vi "App - analyze RUS V6.vi"() -> ()   [LabVIEW 2015] (continued)
"phase"=3.0483689500573607, "Q"=31924.655099131884, "Norm  Ampl"=0.0072958662795648815, "z (inf)"=-0.1566571183741111-0.36129377749056607i, "4corners"={"z (-pi/2)"=-0.47329377749056606+0.020657118374111084i, "z(inf)"=-0.1566571183741111-0.36129377749056607i, "z (pi/2)"=0.22529377749056606-0.044657118374111106i, "z center"=-0.124-0.01200000000000001i, "z(0)"=-0.09134288162588891+0.33729377749056605i, "radius"=0.35081708962667396}}, "timestamp(min)"=939.1499999985099, "timestamp"=timestamp(3493784170 s since 1904-01-01), "Magn Field(T)"=0.0}, {"temperature"=73.253, "lorentzian"={"Amplitude"=0.00019495658027975842, "omega(0)"=663.9104025268014, "Gamma"=0.023023745131469733, "phase"=3.131685954619118, "Q"=28835.89957827249, "Norm  Ampl"=0.011117450646524998, "z (inf)"=0.007216441342229177-0.49484521216169003i, "4corners"={"z (-pi/2)"=-0.47084521216169-0.007216441342229177i, "z(inf)"=0.007216441342229177-0.49484521216169003i, "z (pi/2)"=0.49484521216169003-0.016783558657770845i, "z center"=0.01200000000000001-0.01200000000000001i, "z(0)"=0.016783558657770845+0.47084521216169i, "radius"=0.48286890699329543}}, "timestamp(min)"=940.4833333343267, "timestamp"=timestamp(3493784250 s since 1904-01-01), "Magn Field(T)"=0.0}, {"temperature"=73.185, "lorentzian"={"Amplitude"=0.00017519026701110808, "omega(0)"=663.8919973297286, "Gamma"=0.020890470676565787, "phase"=3.0576685573030025, "Q"=31779.657223063903, "Norm  Ampl"=0.0069963159787889955, "z (inf)"=-0.16807358892896002-0.33772594277637363i, "4corners"={"z (-pi/2)"=-0.47372594277637364+0.02407358892896001i, "z(inf)"=-0.16807358892896002-0.33772594277637363i, "z (pi/2)"=0.19372594277637362-0.03207358892896002i, "z center"=-0.14-0.0040000000000000036i, "z(0)"=-0.11192641107104+0.3297259427763736i, "radius"=0.3349046599815112}}, "timestamp(min)"=941.8000000044703, "timestamp"=timestamp(3493784329 s since 1904-01-01), "Magn Field(T)"=0.0}, {"temperature"=73.117, "lorentzian"={"Amplitude"=0.00017435824596551483, "omega(0)"=663.8725802754554, "Gamma"=0.02068445495091924, "phase"=3.0424021763685554, "Q"=32095.24166098233, "Norm  Ampl"=0.00621721189787517, "z (inf)"=-0.2017652258022671-0.3030966975685784i, "4corners"={"z (-pi/2)"=-0.47109669756857836+0.02576522580226712i, "z(inf)"=-0.2017652258022671-0.3030966975685784i, "z (pi/2)"=0.1270966975685784-0.033765225802267124i, "z center"=-0.172-0.0040000000000000036i, "z(0)"=-0.14223477419773287+0.29509669756857837i, "radius"=0.30057412257792515}}, "timestamp(min)"=943.1166666671634, "timestamp"=timestamp(3493784408 s since 1904-01-01), "Magn Field(T)"=0.0}, {"temperature"=73.048, "lorentzian"={"Amplitude"=0.00017676330015604157, "omega(0)"=663.8531342977661, "Gamma"=0.02121284701140279, "phase"=3.0670891125022886, "Q"=31294.86268113457, "Norm  Ampl"=0.007605974320098498, "z (inf)"=-0.15068891735183343-0.361560422826347i, "4corners"={"z (-pi/2)"=-0.481560422826347+0.02268891735183344i, "z(inf)"=-0.15068891735183343-0.361560422826347i, "z (pi/2)"=0.23356042282634698-0.030688917351833447i, "z center"=-0.124-0.0040000000000000036i, "z(0)"=-0.09731108264816656+0.353560422826347i, "radius"=0.3585550923933016}}, "timestamp(min)"=944.4500000029802, "timestamp"=timestamp(3493784488 s since 1904-01-01), "Magn Field(T)"=0.0}, {"temperature"=72.978, "lorentzian"={"Amplitude"=0.00018345336821167508, "omega(0)"=663.834753319743, "Gamma"=0.022043405813372347, "phase"=3.126951039938785, "Q"=30114.890545499835, "Norm  Ampl"=0.01041417114121995, "z (inf)"=-0.018917026509175042-0.48438865766564027i, "4corners"={"z (-pi/2)"=-0.48438865766564027-0.00508297349082498i, "z(inf)"=-0.018917026509175042-0.48438865766564027i, "z (pi/2)"=0.46038865766564024-0.018917026509175042i, "z center"=-0.01200000000000001-0.01200000000000001i, "z(0)"=-0.00508297349082498+0.46038865766564024i, "radius"=0.47243929678517865}}, "timestamp(min)"=945.7666666656733, "timestamp"=timestamp(3493784567 s since 1904-01-01), "Magn Field(T)"=0.0}, {"temperature"=72.911, "lorentzian"={"Amplitude"=0.0001551220169346823, "omega(0)"=663.8174664217973, "Gamma"=0.018764064565812026, "phase"=3.0713605879648487, "Q"=35377.06151530023, "Norm  Ampl"=0.008325788969481407, "z (inf)"=-0.06713700481821767-0.4546153898054041i, "4corners"={"z (-pi/2)"=-0.4786153898054041+0.01913700481821769i, "z(inf)"=-0.06713700481821767-0.4546153898054041i, "z (pi/2)"=0.4066153898054041-0.04313700481821771i, "z center"=-0.035999999999999976-0.01200000000000001i, "z(0)"=-0.004862995181782275+0.4306153898054041i, "radius"=0.44370924755028435}}, "timestamp(min)"=947.1000000014901, "timestamp"=timestamp(3493784647 s since 1904-01-01), "Magn Field(T)"=0.0}, {"temperature"=72.846, "lorentzian"={"Amplitude"=0.0001555991138381181, "omega(0)"=663.7976768196731, "Gamma"=0.018698213519798536, "phase"=3.053995868272443, "Q"=35500.59347203482, "Norm  Ampl"=0.007017682837638503, "z (inf)"=-0.1408341852026201-0.3778740073328248i, "4corners"={"z (-pi/2)"=-0.48187400733282476+0.028834185202620086i, "z(inf)"=-0.1408341852026201-0.3778740073328248i, "z (pi/2)"=0.2658740073328248-0.03683418520262009i, "z center"=-0.10799999999999998-0.0040000000000000036i, "z(0)"=-0.0751658147973799+0.3698740073328248i, "radius"=0.37531301213390544}}, "timestamp(min)"=948.4166666641831, "timestamp"=timestamp(3493784726 s since 1904-01-01), "Magn Field(T)"=0.0}, {"temperature"=72.777, "lorentzian"={"Amplitude"=0.00015084357573425, "omega(0)"=663.7786903386511, "Gamma"=0.017971078540124134, "phase"=3.0293798474399702, "Q"=36935.94064800443, "Norm  Ampl"=0.005825438199226138, "z (inf)"=-0.19229819911547524-0.3261175918457008i, "4corners"={"z (-pi/2)"=-0.47811759184570085+0.032298199115475205i, "z(inf)"=-0.19229819911547524-0.3261175918457008i, "z (pi/2)"=0.1661175918457008-0.04029819911547521i, "z center"=-0.15600000000000003-0.0040000000000000036i, "z(0)"=-0.11970180088452481+0.3181175918457008i, "radius"=0.32415629291361936}}, "timestamp(min)"=949.7333333343267, "timestamp"=timestamp(3493784805 s since 1904-01-01), "Magn Field(T)"=0.0}, {"temperature"=72.707, "lorentzian"={"Amplitude"=0.00014939699892849853, "omega(0)"=663.7592398477731, "Gamma"=0.017930072072597437, "phase"=3.031276824620436, "Q"=37019.329156082844, "Norm  Ampl"=0.006595607315274654, "z (inf)"=-0.15649760753219724-0.3696156584222518i, "4corners"={"z (-pi/2)"=-0.4816156584222518+0.036497607532197246i, "z(inf)"=-0.15649760753219724-0.3696156584222518i, "z (pi/2)"=0.2496156584222518-0.04449760753219725i, "z center"=-0.11599999999999999-0.0040000000000000036i, "z(0)"=-0.07550239246780274+0.3616156584222518i, "radius"=0.36785169008632895}}, "timestamp(min)"=951.0666666701436, "timestamp"=timestamp(3493784885 s since 1904-01-01), "Magn Field(T)"=0.0}, {"temperature"=72.643, "lorentzian"={"Amplitude"=0.00017077398769670094, "omega(0)"=663.738826060015, "Gamma"=0.020607074561124927, "phase"=3.0746062633397298, "Q"=32209.269884050045, "Norm  Ampl"=0.0086712605421239, "z (inf)"=-0.08816615902804703-0.43184674010553753i, "4corners"={"z (-pi/2)"=-0.4798467401055375+0.01616615902804702i, "z(inf)"=-0.08816615902804703-0.43184674010553753i, "z (pi/2)"=0.3598467401055375-0.040166159028047044i, "z center"=-0.06-0.01200000000000001i, "z(0)"=-0.031833840971952965+0.4078467401055375i, "radius"=0.4207904676815291}}, "timestamp(min)"=952.3833333328366, "timestamp"=timestamp(3493784964 s since 1904-01-01), "Magn Field(T)"=0.0}, {"temperature"=72.574, "lorentzian"={"Amplitude"=0.00015213404269060979, "omega(0)"=663.7213392465111, "Gamma"=0.01837305169166479, "phase"=3.035741424854037, "Q"=36124.719528635425, "Norm  Ampl"=0.006585091339083578, "z (inf)"=-0.16186736619318068-0.3604042931463336i, "4corners"={"z (-pi/2)"=-0.4804042931463336+0.033867366193180676i, "z(inf)"=-0.16186736619318068-0.3604042931463336i, "z (pi/2)"=0.2324042931463336-0.04186736619318068i, "z center"=-0.124-0.0040000000000000036i, "z(0)"=-0.08613263380681932+0.3524042931463336i, "radius"=0.3584103201577016}}, "timestamp(min)"=953.7000000029802, "timestamp"=timestamp(3493785043 s since 1904-01-01), "Magn Field(T)"=0.0}, {"temperature"=72.507, "lorentzian"={"Amplitude"=0.0001470715960104401, "omega(0)"=663.7025470782887, "Gamma"=0.01782665731894476, "phase"=3.04998161802813, "Q"=37230.90286662762, "Norm  Ampl"=0.006247681308114839, "z (inf)"=-0.16406188847504188-0.35299883018424616i, "4corners"={"z (-pi/2)"=-0.48099883018424616+0.028061888475041874i, "z(inf)"=-0.16406188847504188-0.35299883018424616i, "z (pi/2)"=0.21699883018424615-0.03606188847504188i, "z center"=-0.132-0.0040000000000000036i, "z(0)"=-0.09993811152495813+0.34499883018424615i, "radius"=0.35046846956974365}}, "timestamp(min)"=955.0333333313465, "timestamp"=timestamp(3493785123 s since 1904-01-01), "Magn Field(T)"=0.0}, {"temperature"=72.439, "lorentzian"={"Amplitude"=0.0001556972144457539, "omega(0)"=663.6810373710007, "Gamma"=0.0190413758844246, "phase"=3.0950823081436862, "Q"=34854.67864293758, "Norm  Ampl"=0.006603870241185977, "z (inf)"=-0.15612475706680048-0.35044181083865616i, "4corners"={"z (-pi/2)"=-0.4864418108386562+0.012124757066800471i, "z(inf)"=-0.15612475706680048-0.35044181083865616i, "z (pi/2)"=0.20644181083865615-0.02012475706680048i, "z center"=-0.14-0.0040000000000000036i, "z(0)"=-0.12387524293319954+0.34244181083865616i, "radius"=0.3468168624614878}}, "timestamp(min)"=956.3500000014901, "timestamp"=timestamp(3493785202 s since 1904-01-01), "Magn Field(T)"=0.0}, {"temperature"=72.371, "lorentzian"={"Amplitude"=0.0001507592891099395, "omega(0)"=663.6638983583827, "Gamma"=0.01869568647863634, "phase"=3.0980461327038666, "Q"=35498.23640425052, "Norm  Ampl"=0.006397856598824616, "z (inf)"=-0.14689735890560787-0.35388589109003726i, "4corners"={"z (-pi/2)"=-0.47388589109003726+0.002897358905607862i, "z(inf)"=-0.14689735890560787-0.35388589109003726i, "z (pi/2)"=0.20988589109003725-0.026897358905607884i, "z center"=-0.132-0.01200000000000001i, "z(0)"=-0.11710264109439214+0.32988589109003724i, "radius"=0.3422103064327422}}, "timestamp(min)"=957.683333337307, "timestamp"=timestamp(3493785282 s since 1904-01-01), "Magn Field(T)"=0.0}, {"temperature"=72.308, "lorentzian"={"Amplitude"=0.00016230426236795705, "omega(0)"=663.6439303978735, "Gamma"=0.01982415794364744, "phase"=3.131202541165063, "Q"=33476.5255747236, "Norm  Ampl"=0.008567093112471861, "z (inf)"=-0.05649004993272625-0.4441308735094935i, "4corners"={"z (-pi/2)"=-0.48413087350949346-0.00750995006727375i, "z(inf)"=-0.05649004993272625-0.4441308735094935i, "z (pi/2)"=0.3801308735094935-0.01649004993272627i, "z center"=-0.05199999999999999-0.01200000000000001i, "z(0)"=-0.04750995006727373+0.42013087350949346i, "radius"=0.4321541997811386}}, "timestamp(min)"=959.0, "timestamp"=timestamp(3493785361 s since 1904-01-01), "Magn Field(T)"=0.0}, {"temperature"=72.238, "lorentzian"={"Amplitude"=0.0001587208237648037, "omega(0)"=663.6241437684071, "Gamma"=0.018918376740188685, "phase"=3.0783676700778537, "Q"=35078.281444657834, "Norm  Ampl"=0.006359561424550766, "z (inf)"=-0.16123941943617293-0.34748622561900455i, "4corners"={"z (-pi/2)"=-0.47548622561900455+0.009239419436172912i, "z(inf)"=-0.16123941943617293-0.34748622561900455i, "z (pi/2)"=0.19548622561900453-0.03323941943617294i, "z center"=-0.14-0.01200000000000001i, "z(0)"=-0.11876058056382709+0.32348622561900453i, "radius"=0.33615788034504157}}, "timestamp(min)"=960.3166666701436, "timestamp"=timestamp(3493785440 s since 1904-01-01), "Magn Field(T)"=0.0}, {"temperature"=72.173, "lorentzian"={"Amplitude"=0.00014945097138632582, "omega(0)"=663.6053258833265, "Gamma"=0.017943141405183435, "phase"=3.0710983273781256, "Q"=36983.78733679396, "Norm  Ampl"=0.006165904771094313, "z (inf)"=-0.1562043116839784-0.35478225857476353i, "4corners"={"z (-pi/2)"=-0.4747822585747635+0.012204311683978373i, "z(inf)"=-0.1562043116839784-0.35478225857476353i, "z (pi/2)"=0.21078225857476351-0.03620431168397839i, "z center"=-0.132-0.01200000000000001i, "z(0)"=-0.10779568831602163+0.3307822585747635i, "radius"=0.3436357453724964}}, "timestamp(min)"=961.6499999985099, "timestamp"=timestamp(3493785520 s since 1904-01-01), "Magn Field(T)"=0.0}, {"temperature"=72.106, "lorentzian"={"Amplitude"=0.00014166531123358068, "omega(0)"=663.5880613487568, "Gamma"=0.017621215492130873, "phase"=3.063673431163844, "Q"=37658.47263176006, "Norm  Ampl"=0.007707115263841109, "z (inf)"=-0.07804560451196209-0.45604997580422607i, "4corners"={"z (-pi/2)"=-0.48004997580422604+0.014045604511962087i, "z(inf)"=-0.07804560451196209-0.45604997580422607i, "z (pi/2)"=0.39204997580422607-0.05404560451196212i, "z center"=-0.043999999999999984-0.020000000000000018i, "z(0)"=-0.009954395488037879+0.41604997580422604i, "radius"=0.43737705082165784}}, "timestamp(min)"=962.9666666686535, "timestamp"=timestamp(3493785599 s since 1904-01-01), "Magn Field(T)"=0.0}, {"temperature"=72.039, "lorentzian"={"Amplitude"=0.00010361030809420268, "omega(0)"=663.5698546355719, "Gamma"=0.016439285091381955, "phase"=3.1094946906609193, "Q"=40364.885148408204, "Norm  Ampl"=0.005333823694357822, "z (inf)"=-0.1584125865349883-0.38428881406653514i, "4corners"={"z (-pi/2)"=-0.47228881406653517-0.04958741346501172i, "z(inf)"=-0.1584125865349883-0.38428881406653514i, "z (pi/2)"=0.17628881406653513-0.07041258653498828i, "z center"=-0.14800000000000002-0.06i, "z(0)"=-0.13758741346501174+0.26428881406653515i, "radius"=0.32445593982392806}}, "timestamp(min)"=964.2833333313465, "timestamp"=timestamp(3493785678 s since 1904-01-01), "Magn Field(T)"=0.0}, {"temperature"=71.974, "lorentzian"={"Amplitude"=0.0001353918285003591, "omega(0)"=663.5515429002106, "Gamma"=0.016337688977960896, "phase"=3.1152659157247515, "Q"=40614.773839514506, "Norm  Ampl"=0.0059967070933330206, "z (inf)"=-0.11766204581152509-0.37892025850284383i, "4corners"={"z (-pi/2)"=-0.4749202585028438-0.0023379541884749073i, "z(inf)"=-0.11766204581152509-0.37892025850284383i, "z (pi/2)"=0.25892025850284384-0.021662045811525116i, "z center"=-0.10799999999999998-0.01200000000000001i, "z(0)"=-0.09833795418847488+0.3549202585028438i, "radius"=0.36704745092298047}}, "timestamp(min)"=965.6166666671634, "timestamp"=timestamp(3493785758 s since 1904-01-01), "Magn Field(T)"=0.0}, {"temperature"=71.908, "lorentzian"={"Amplitude"=0.00020447876795810522, "omega(0)"=663.5338391109882, "Gamma"=0.024406535860778355, "phase"=3.462541685023603, "Q"=27186.727477261382, "Norm  Ampl"=0.009353380375411984, "z (inf)"=0.028897345607210093-0.415663392708284i, "4corners"={"z (-pi/2)"=-0.45566339270828404-0.1728973456072101i, "z(inf)"=0.028897345607210093-0.415663392708284i, "z (pi/2)"=0.271663392708284+0.06889734560721013i, "z center"=-0.09200000000000003-0.05199999999999999i, "z(0)"=-0.21289734560721013+0.311663392708284i, "radius"=0.3832326073952591}}, "timestamp(min)"=966.933333337307, "timestamp"=timestamp(3493785837 s since 1904-01-01), "Magn Field(T)"=0.0}, {"temperature"=71.842, "lorentzian"={"Amplitude"=0.00020284598772034006, "omega(0)"=663.5159545204048, "Gamma"=0.02385301531569419, "phase"=3.438102919866405, "Q"=27816.858612581433, "Norm  Ampl"=0.010641694016462908, "z (inf)"=0.09435410712337688-0.502667705428403i, "4corners"={"z (-pi/2)"=-0.462667705428403-0.20635410712337687i, "z(inf)"=0.09435410712337688-0.502667705428403i, "z (pi/2)"=0.39066770542840307+0.05435410712337685i, "z center"=-0.035999999999999976-0.07600000000000001i, "z(0)"=-0.16635410712337684+0.35066770542840303i, "radius"=0.4461362169780339}}, "timestamp(min)"=968.2666666656733, "timestamp"=timestamp(3493785917 s since 1904-01-01), "Magn Field(T)"=0.0}, {"temperature"=71.776, "lorentzian"={"Amplitude"=0.0001158178599625776, "omega(0)"=663.4970989685446, "Gamma"=0.017705924903385337, "phase"=3.1260543468802098, "Q"=37473.168026465835, "Norm  Ampl"=0.006876638691775869, "z (inf)"=-0.09003453488478114-0.45633376972380324i, "4corners"={"z (-pi/2)"=-0.47233376972380325-0.06196546511521888i, "z(inf)"=-0.09003453488478114-0.45633376972380324i, "z (pi/2)"=0.3043337697238032-0.07403453488478112i, "z center"=-0.08400000000000002-0.068i, "z(0)"=-0.0779654651152189+0.32033376972380323i, "radius"=0.3883806538940572}}, "timestamp(min)"=969.5833333358169, "timestamp"=timestamp(3493785996 s since 1904-01-01), "Magn Field(T)"=0.0}, {"temperature"=71.708, "lorentzian"={"Amplitude"=0.00014344606787871066, "omega(0)"=663.4769127694987, "Gamma"=0.018079577085066488, "phase"=3.0739753162348773, "Q"=36697.59030577781, "Norm  Ampl"=0.007230938052613988, "z (inf)"=-0.1030229929735954-0.4110366596727773i, "4corners"={"z (-pi/2)"=-0.4750366596727773+0.01502299297359539i, "z(inf)"=-0.1030229929735954-0.4110366596727773i, "z (pi/2)"=0.3230366596727773-0.03902299297359541i, "z center"=-0.07600000000000001-0.01200000000000001i, "z(0)"=-0.04897700702640461+0.3870366596727773i, "radius"=0.3999506193420119}}, "timestamp(min)"=970.8999999985099, "timestamp"=timestamp(3493786075 s since 1904-01-01), "Magn Field(T)"=0.0}, {"temperature"=71.643, "lorentzian"={"Amplitude"=1.7606488630633843e-05, "omega(0)"=663.4981912028674, "Gamma"=0.002347216628142593, "phase"=2.6632845873121296, "Q"=282674.4592926256, "Norm  Ampl"=0.0022609898934732864, "z (inf)"=-0.0153691348783212-0.3791618846869318i, "4corners"={"z (-pi/2)"=-0.4271618846869317+0.9193691348783213i, "z(inf)"=-0.0153691348783212-0.3791618846869318i, "z (pi/2)"=1.283161884686932+0.03263086512167873i, "z center"=0.42800000000000005+0.476i, "z(0)"=0.8713691348783212+1.3311618846869318i, "radius"=0.9632642621752642}}, "timestamp(min)"=972.2333333343267, "timestamp"=timestamp(3493786155 s since 1904-01-01), "Magn Field(T)"=0.0}, {"temperature"=71.578, "lorentzian"={"Amplitude"=1.4211102692804694e-05, "omega(0)"=663.499400259395, "Gamma"=0.0015188613859837142, "phase"=3.0098558230419314, "Q"=436839.99500037933, "Norm  Ampl"=0.0014038362866800934, "z (inf)"=0.3705916271616414-0.5202603006819091i, "4corners"={"z (-pi/2)"=-0.4242603006819091+0.5174083728383586i, "z(inf)"=0.3705916271616414-0.5202603006819091i, "z (pi/2)"=1.408260300681909+0.2745916271616414i, "z center"=0.492+0.396i, "z(0)"=0.6134083728383586+1.3122603006819091i, "radius"=0.9242688632648837}}, "timestamp(min)"=973.5500000044703, "timestamp"=timestamp(3493786234 s since 1904-01-01), "Magn Field(T)"=0.0}, {"temperature"=71.514, "lorentzian"={"Amplitude"=0.0010685633366742913, "omega(0)"=663.450380905746, "Gamma"=0.15922878254567352, "phase"=4.5585256955829605, "Q"=4166.648581360851, "Norm  Ampl"=0.08739969324990009, "z (inf)"=0.322409387202908+0.12787822949289898i, "4corners"={"z (-pi/2)"=-0.304121770507101-0.330409387202908i, "z(inf)"=0.322409387202908+0.12787822949289898i, "z (pi/2)"=-0.135878229492899+0.754409387202908i, "z center"=-0.21999999999999997+0.21199999999999997i, "z(0)"=-0.762409387202908+0.296121770507101i, "radius"=0.5488938108587886}}, "timestamp(min)"=974.8833333328366, "timestamp"=timestamp(3493786314 s since 1904-01-01), "Magn Field(T)"=0.0}, {"temperature"=71.446, "lorentzian"={"Amplitude"=0.0029607355721983555, "omega(0)"=663.468044758759, "Gamma"=0.47900225843268496, "phase"=-0.5808048204263985, "Q"=1385.104210008641, "Norm  Ampl"=0.30913694678107567, "z (inf)"=0.10211629149371892+0.7595487666345311i, "4corners"={"z (-pi/2)"=0.2875487666345311-0.13411629149371895i, "z(inf)"=0.10211629149371892+0.7595487666345311i, "z (pi/2)"=-0.7915487666345311+0.5741162914937189i, "z center"=-0.252+0.21999999999999997i, "z(0)"=-0.6061162914937189-0.31954876663453113i, "radius"=0.6453768042609745}}, "timestamp(min)"=976.2000000029802, "timestamp"=timestamp(3493786393 s since 1904-01-01), "Magn Field(T)"=0.0}, {"temperature"=71.383, "lorentzian"={"Amplitude"=0.0010611794064622126, "omega(0)"=663.4473219222272, "Gamma"=0.2080875040394991, "phase"=-1.3216612968573798, "Q"=3188.309288366935, "Norm  Ampl"=0.11037021324273609, "z (inf)"=0.31802725973655793+0.294779205449031i, "4corners"={"z (-pi/2)"=-0.06522079455096902-0.3500272597365579i, "z(inf)"=0.31802725973655793+0.294779205449031i, "z (pi/2)"=-0.326779205449031+0.678027259736558i, "z center"=-0.196+0.16400000000000003i, "z(0)"=-0.710027259736558+0.033220794550969046i, "radius"=0.5304028886894891}}, "timestamp(min)"=977.5166666656733, "timestamp"=timestamp(3493786472 s since 1904-01-01), "Magn Field(T)"=0.0}, {"temperature"=71.316, "lorentzian"={"Amplitude"=0.003475248520660529, "omega(0)"=663.321849078867, "Gamma"=0.42900679763503213, "phase"=-1.1532083704249727, "Q"=1546.1802767124755, "Norm  Ampl"=0.3966685315298843, "z (inf)"=0.3771678036337911+0.7869862344056386i, "4corners"={"z (-pi/2)"=-0.09301376559436136-0.43316780363379104i, "z(inf)"=0.3771678036337911+0.7869862344056386i, "z (pi/2)"=-0.8429862344056386+1.257167803633791i, "z center"=-0.46799999999999997+0.41200000000000003i, "z(0)"=-1.313167803633791+0.037013765594361425i, "radius"=0.924620620737439}}, "timestamp(min)"=978.8500000014901, "timestamp"=timestamp(3493786552 s since 1904-01-01), "Magn Field(T)"=0.0}, {"temperature"=71.25, "lorentzian"={"Amplitude"=0.0, "omega(0)"=0.0, "Gamma"=0.0, "phase"=0.0, "Q"=0.0, "Norm  Ampl"=0.0, "z (inf)"=0.0+0.0i, "4corners"={"z (-pi/2)"=0.0+0.0i, "z(inf)"=0.0+0.0i, "z (pi/2)"=0.0+0.0i, "z center"=0.0+0.0i, "z(0)"=0.0+0.0i, "radius"=0.0}}, "timestamp(min)"=980.1666666641831, "timestamp"=timestamp(3493786631 s since 1904-01-01), "Magn Field(T)"=0.0}, {"temperature"=71.184, "lorentzian"={"Amplitude"=0.003475248520660529, "omega(0)"=663.321849078867, "Gamma"=0.42900679763503213, "phase"=-1.1532083704249727, "Q"=1546.1802767124755, "Norm  Ampl"=0.3966685315298843, "z (inf)"=0.3771678036337911+0.7869862344056386i, "4corners"={"z (-pi/2)"=-0.09301376559436136-0.43316780363379104i, "z(inf)"=0.3771678036337911+0.7869862344056386i, "z (pi/2)"=-0.8429862344056386+1.257167803633791i, "z center"=-0.46799999999999997+0.41200000000000003i, "z(0)"=-1.313167803633791+0.037013765594361425i, "radius"=0.924620620737439}}, "timestamp(min)"=981.4833333343267, "timestamp"=timestamp(3493786710 s since 1904-01-01), "Magn Field(T)"=0.0}, {"temperature"=71.122, "lorentzian"={"Amplitude"=0.0, "omega(0)"=0.0, "Gamma"=0.0, "phase"=0.0, "Q"=0.0, "Norm  Ampl"=0.0, "z (inf)"=0.0+0.0i, "4corners"={"z (-pi/2)"=0.0+0.0i, "z(inf)"=0.0+0.0i, "z (pi/2)"=0.0+0.0i, "z center"=0.0+0.0i, "z(0)"=0.0+0.0i, "radius"=0.0}}, "timestamp(min)"=982.8166666701436, "timestamp"=timestamp(3493786790 s since 1904-01-01), "Magn Field(T)"=0.0}, {"temperature"=71.056, "lorentzian"={"Amplitude"=0.0, "omega(0)"=0.0, "Gamma"=0.0, "phase"=0.0, "Q"=0.0, "Norm  Ampl"=0.0, "z (inf)"=0.0+0.0i, "4corners"={"z (-pi/2)"=0.0+0.0i, "z(inf)"=0.0+0.0i, "z (pi/2)"=0.0+0.0i, "z center"=0.0+0.0i, "z(0)"=0.0+0.0i, "radius"=0.0}}, "timestamp(min)"=984.1333333328366, "timestamp"=timestamp(3493786869 s since 1904-01-01), "Magn Field(T)"=0.0}, {"temperature"=70.993, "lorentzian"={"Amplitude"=0.0, "omega(0)"=0.0, "Gamma"=0.0, "phase"=0.0, "Q"=0.0, "Norm  Ampl"=0.0, "z (inf)"=0.0+0.0i, "4corners"={"z (-pi/2)"=0.0+0.0i, "z(inf)"=0.0+0.0i, "z (pi/2)"=0.0+0.0i, "z center"=0.0+0.0i, "z(0)"=0.0+0.0i, "radius"=0.0}}, "timestamp(min)"=985.4666666686535, "timestamp"=timestamp(3493786949 s since 1904-01-01), "Magn Field(T)"=0.0}, {"temperature"=70.928, "lorentzian"={"Amplitude"=0.0, "omega(0)"=0.0, "Gamma"=0.0, "phase"=0.0, "Q"=0.0, "Norm  Ampl"=0.0, "z (inf)"=0.0+0.0i, "4corners"={"z (-pi/2)"=0.0+0.0i, "z(inf)"=0.0+0.0i, "z (pi/2)"=0.0+0.0i, "z center"=0.0+0.0i, "z(0)"=0.0+0.0i, "radius"=0.0}}, "timestamp(min)"=986.7833333313465, "timestamp"=timestamp(3493787028 s since 1904-01-01), "Magn Field(T)"=0.0}, {"temperature"=70.86, "lorentzian"={"Amplitude"=0.0, "omega(0)"=0.0, "Gamma"=0.0, "phase"=0.0, "Q"=0.0, "Norm  Ampl"=0.0, "z (inf)"=0.0+0.0i, "4corners"={"z (-pi/2)"=0.0+0.0i, "z(inf)"=0.0+0.0i, "z (pi/2)"=0.0+0.0i, "z center"=0.0+0.0i, "z(0)"=0.0+0.0i, "radius"=0.0}}, "timestamp(min)"=988.1000000014901, "timestamp"=timestamp(3493787107 s since 1904-01-01), "Magn Field(T)"=0.0}, {"temperature"=70.8, "lorentzian"={"Amplitude"=0.0, "omega(0)"=0.0, "Gamma"=0.0, "phase"=0.0, "Q"=0.0, "Norm  Ampl"=0.0, "z (inf)"=0.0+0.0i, "4corners"={"z (-pi/2)"=0.0+0.0i, "z(inf)"=0.0+0.0i, "z (pi/2)"=0.0+0.0i, "z center"=0.0+0.0i, "z(0)"=0.0+0.0i, "radius"=0.0}}, "timestamp(min)"=989.433333337307, "timestamp"=timestamp(3493787187 s since 1904-01-01), "Magn Field(T)"=0.0}, {"temperature"=70.734, "lorentzian"={"Amplitude"=0.00014741895752361318, "omega(0)"=663.2012958301423, "Gamma"=0.019526191075777525, "phase"=3.133366552808286, "Q"=33964.703779471434, "Norm  Ampl"=0.006276995745365551, "z (inf)"=-0.15864437734220443-0.3334545706341914i, "4corners"={"z (-pi/2)"=-0.47745457063419144-0.009355622657795592i, "z(inf)"=-0.15864437734220443-0.3334545706341914i, "z (pi/2)"=0.1654545706341914-0.01464437734220443i, "z center"=-0.15600000000000003-0.01200000000000001i, "z(0)"=-0.15335562265779562+0.3094545706341914i, "radius"=0.3214654471527855}}, "timestamp(min)"=990.75, "timestamp"=timestamp(3493787266 s since 1904-01-01), "Magn Field(T)"=0.0}, {"temperature"=70.67, "lorentzian"={"Amplitude"=0.0, "omega(0)"=0.0, "Gamma"=0.0, "phase"=0.0, "Q"=0.0, "Norm  Ampl"=0.0, "z (inf)"=0.0+0.0i, "4corners"={"z (-pi/2)"=0.0+0.0i, "z(inf)"=0.0+0.0i, "z (pi/2)"=0.0+0.0i, "z center"=0.0+0.0i, "z(0)"=0.0+0.0i, "radius"=0.0}}, "timestamp(min)"=992.0833333358169, "timestamp"=timestamp(3493787346 s since 1904-01-01), "Magn Field(T)"=0.0}, {"temperature"=70.607, "lorentzian"={"Amplitude"=0.00015328744837051362, "omega(0)"=663.1800332004171, "Gamma"=0.020013063108302323, "phase"=3.144815040514048, "Q"=33137.35781532114, "Norm  Ampl"=0.006378181417753034, "z (inf)"=-0.1629730241332717-0.322699255004469i, "4corners"={"z (-pi/2)"=-0.482699255004469-0.005026975866728277i, "z(inf)"=-0.1629730241332717-0.322699255004469i, "z (pi/2)"=0.15469925500446902-0.00297302413327173i, "z center"=-0.16399999999999998-0.0040000000000000036i, "z(0)"=-0.16502697586672826+0.314699255004469i, "radius"=0.31870090966270304}}, "timestamp(min)"=993.3999999985099, "timestamp"=timestamp(3493787425 s since 1904-01-01), "Magn Field(T)"=0.0}, {"temperature"=70.54, "lorentzian"={"Amplitude"=0.00016009520963442775, "omega(0)"=663.1586234942882, "Gamma"=0.021315116129614096, "phase"=3.2383816283953406, "Q"=31112.128100157555, "Norm  Ampl"=0.00921059739114969, "z (inf)"=-0.01824123099103222-0.4340932765652777i, "4corners"={"z (-pi/2)"=-0.4900932765652777-0.04575876900896778i, "z(inf)"=-0.01824123099103222-0.4340932765652777i, "z (pi/2)"=0.3700932765652777+0.037758769008967775i, "z center"=-0.06-0.0040000000000000036i, "z(0)"=-0.10175876900896777+0.4260932765652777i, "radius"=0.4321157499279571}}, "timestamp(min)"=994.7166666686535, "timestamp"=timestamp(3493787504 s since 1904-01-01), "Magn Field(T)"=0.0}, {"temperature"=70.48, "lorentzian"={"Amplitude"=0.0, "omega(0)"=0.0, "Gamma"=0.0, "phase"=0.0, "Q"=0.0, "Norm  Ampl"=0.0, "z (inf)"=0.0+0.0i, "4corners"={"z (-pi/2)"=0.0+0.0i, "z(inf)"=0.0+0.0i, "z (pi/2)"=0.0+0.0i, "z center"=0.0+0.0i, "z(0)"=0.0+0.0i, "radius"=0.0}}, "timestamp(min)"=996.0500000044703, "timestamp"=timestamp(3493787584 s since 1904-01-01), "Magn Field(T)"=0.0}, {"temperature"=70.414, "lorentzian"={"Amplitude"=0.00018369885854043977, "omega(0)"=663.1389266485459, "Gamma"=0.0282063915207932, "phase"=3.3512799945839324, "Q"=23510.23618741493, "Norm  Ampl"=0.011412554723516653, "z (inf)"=0.04022098408390162-0.471746283827637i, "4corners"={"z (-pi/2)"=-0.439746283827637-0.16022098408390162i, "z(inf)"=0.04022098408390162-0.471746283827637i, "z (pi/2)"=0.351746283827637+0.008220984083901595i, "z center"=-0.043999999999999984-0.07600000000000001i, "z(0)"=-0.1282209840839016+0.319746283827637i, "radius"=0.4046088176540959}}, "timestamp(min)"=997.3666666671634, "timestamp"=timestamp(3493787663 s since 1904-01-01), "Magn Field(T)"=0.0}, {"temperature"=70.35, "lorentzian"={"Amplitude"=0.0, "omega(0)"=0.0, "Gamma"=0.0, "phase"=0.0, "Q"=0.0, "Norm  Ampl"=0.0, "z (inf)"=0.0+0.0i, "4corners"={"z (-pi/2)"=0.0+0.0i, "z(inf)"=0.0+0.0i, "z (pi/2)"=0.0+0.0i, "z center"=0.0+0.0i, "z(0)"=0.0+0.0i, "radius"=0.0}}, "timestamp(min)"=998.683333337307, "timestamp"=timestamp(3493787742 s since 1904-01-01), "Magn Field(T)"=0.0}, {"temperature"=70.285, "lorentzian"={"Amplitude"=0.00013372585951176968, "omega(0)"=663.1015876451874, "Gamma"=0.017494743955420233, "phase"=3.1270308468041366, "Q"=37902.9032568233, "Norm  Ampl"=0.005528544947343909, "z (inf)"=-0.16860153966316427-0.31997826285810693i, "4corners"={"z (-pi/2)"=-0.4799782628581069+0.0006015396631642873i, "z(inf)"=-0.16860153966316427-0.31997826285810693i, "z (pi/2)"=0.15197826285810695-0.008601539663164294i, "z center"=-0.16399999999999998-0.0040000000000000036i, "z(0)"=-0.1593984603368357+0.3119782628581069i, "radius"=0.3160117668158871}}, "timestamp(min)"=1000.0166666656733, "timestamp"=timestamp(3493787822 s since 1904-01-01), "Magn Field(T)"=0.0}, {"temperature"=70.221, "lorentzian"={"Amplitude"=0.0, "omega(0)"=0.0, "Gamma"=0.0, "phase"=0.0, "Q"=0.0, "Norm  Ampl"=0.0, "z (inf)"=0.0+0.0i, "4corners"={"z (-pi/2)"=0.0+0.0i, "z(inf)"=0.0+0.0i, "z (pi/2)"=0.0+0.0i, "z center"=0.0+0.0i, "z(0)"=0.0+0.0i, "radius"=0.0}}, "timestamp(min)"=1001.3333333358169, "timestamp"=timestamp(3493787901 s since 1904-01-01), "Magn Field(T)"=0.0}, {"temperature"=70.16, "lorentzian"={"Amplitude"=0.00013178769772944474, "omega(0)"=663.0600120819944, "Gamma"=0.017472911437437226, "phase"=3.188536216441653, "Q"=37947.883754583156, "Norm  Ampl"=0.007843067538654333, "z (inf)"=-0.030936176529874185-0.4443756056972315i, "4corners"={"z (-pi/2)"=-0.5003756056972315-0.0170638234701258i, "z(inf)"=-0.030936176529874185-0.4443756056972315i, "z (pi/2)"=0.3963756056972315+0.02506382347012581i, "z center"=-0.05199999999999999+0.0040000000000000036i, "z(0)"=-0.0730638234701258+0.4523756056972315i, "radius"=0.44887010197109345}}, "timestamp(min)"=1002.6666666641831, "timestamp"=timestamp(3493787981 s since 1904-01-01), "Magn Field(T)"=0.0}, {"temperature"=70.095, "lorentzian"={"Amplitude"=0.0, "omega(0)"=0.0, "Gamma"=0.0, "phase"=0.0, "Q"=0.0, "Norm  Ampl"=0.0, "z (inf)"=0.0+0.0i, "4corners"={"z (-pi/2)"=0.0+0.0i, "z(inf)"=0.0+0.0i, "z (pi/2)"=0.0+0.0i, "z center"=0.0+0.0i, "z(0)"=0.0+0.0i, "radius"=0.0}}, "timestamp(min)"=1003.9833333343267, "timestamp"=timestamp(3493788060 s since 1904-01-01), "Magn Field(T)"=0.0}, {"temperature"=70.033, "lorentzian"={"Amplitude"=0.00012375909360109864, "omega(0)"=663.0228973120825, "Gamma"=0.01623350977553243, "phase"=3.088013688124358, "Q"=40842.85570280112, "Norm  Ampl"=0.005522235415342656, "z (inf)"=-0.1582175095241022-0.3436869211707823i, "4corners"={"z (-pi/2)"=-0.4796869211707823+0.014217509524102185i, "z(inf)"=-0.1582175095241022-0.3436869211707823i, "z (pi/2)"=0.1996869211707823-0.022217509524102192i, "z center"=-0.14-0.0040000000000000036i, "z(0)"=-0.12178249047589783+0.3356869211707823i, "radius"=0.34017507561217064}}, "timestamp(min)"=1005.3000000044703, "timestamp"=timestamp(3493788139 s since 1904-01-01), "Magn Field(T)"=0.0}, {"temperature"=69.969, "lorentzian"={"Amplitude"=0.0, "omega(0)"=0.0, "Gamma"=0.0, "phase"=0.0, "Q"=0.0, "Norm  Ampl"=0.0, "z (inf)"=0.0+0.0i, "4corners"={"z (-pi/2)"=0.0+0.0i, "z(inf)"=0.0+0.0i, "z (pi/2)"=0.0+0.0i, "z center"=0.0+0.0i, "z(0)"=0.0+0.0i, "radius"=0.0}}, "timestamp(min)"=1006.6333333328366, "timestamp"=timestamp(3493788219 s since 1904-01-01), "Magn Field(T)"=0.0}, {"temperature"=69.905, "lorentzian"={"Amplitude"=0.00012659811730030067, "omega(0)"=662.9654599727345, "Gamma"=0.016725252746731926, "phase"=3.17432731164591, "Q"=39638.591416938456, "Norm  Ampl"=0.00789842824763509, "z (inf)"=-0.004543960045143939-0.46799267680432916i, "4corners"={"z (-pi/2)"=-0.4919926768043292-0.011456039954856076i, "z(inf)"=-0.004543960045143939-0.46799267680432916i, "z (pi/2)"=0.45199267680432914+0.019456039954856084i, "z center"=-0.020000000000000018+0.0040000000000000036i, "z(0)"=-0.0354560399548561+0.47599267680432916i, "radius"=0.47224567348785956}}, "timestamp(min)"=1007.9500000029802, "timestamp"=timestamp(3493788298 s since 1904-01-01), "Magn Field(T)"=0.0}, {"temperature"=69.845, "lorentzian"={"Amplitude"=0.00012659811730030067, "omega(0)"=662.9654599727345, "Gamma"=0.016725252746731926, "phase"=3.17432731164591, "Q"=39638.591416938456, "Norm  Ampl"=0.00789842824763509, "z (inf)"=-0.004543960045143939-0.46799267680432916i, "4corners"={"z (-pi/2)"=-0.4919926768043292-0.011456039954856076i, "z(inf)"=-0.004543960045143939-0.46799267680432916i, "z (pi/2)"=0.45199267680432914+0.019456039954856084i, "z center"=-0.020000000000000018+0.0040000000000000036i, "z(0)"=-0.0354560399548561+0.47599267680432916i, "radius"=0.47224567348785956}}, "timestamp(min)"=1009.2833333313465, "timestamp"=timestamp(3493788378 s since 1904-01-01), "Magn Field(T)"=0.0}, {"temperature"=69.78, "lorentzian"={"Amplitude"=0.0, "omega(0)"=0.0, "Gamma"=0.0, "phase"=0.0, "Q"=0.0, "Norm  Ampl"=0.0, "z (inf)"=0.0+0.0i, "4corners"={"z (-pi/2)"=0.0+0.0i, "z(inf)"=0.0+0.0i, "z (pi/2)"=0.0+0.0i, "z center"=0.0+0.0i, "z(0)"=0.0+0.0i, "radius"=0.0}}, "timestamp(min)"=1010.6000000014901, "timestamp"=timestamp(3493788457 s since 1904-01-01), "Magn Field(T)"=0.0}, {"temperature"=69.717, "lorentzian"={"Amplitude"=0.0, "omega(0)"=0.0, "Gamma"=0.0, "phase"=0.0, "Q"=0.0, "Norm  Ampl"=0.0, "z (inf)"=0.0+0.0i, "4corners"={"z (-pi/2)"=0.0+0.0i, "z(inf)"=0.0+0.0i, "z (pi/2)"=0.0+0.0i, "z center"=0.0+0.0i, "z(0)"=0.0+0.0i, "radius"=0.0}}, "timestamp(min)"=1011.9166666641831, "timestamp"=timestamp(3493788536 s since 1904-01-01), "Magn Field(T)"=0.0}, {"temperature"=69.656, "lorentzian"={"Amplitude"=0.0, "omega(0)"=0.0, "Gamma"=0.0, "phase"=0.0, "Q"=0.0, "Norm  Ampl"=0.0, "z (inf)"=0.0+0.0i, "4corners"={"z (-pi/2)"=0.0+0.0i, "z(inf)"=0.0+0.0i, "z (pi/2)"=0.0+0.0i, "z center"=0.0+0.0i, "z(0)"=0.0+0.0i, "radius"=0.0}}, "timestamp(min)"=1013.25, "timestamp"=timestamp(3493788616 s since 1904-01-01), "Magn Field(T)"=0.0}, {"temperature"=69.592, "lorentzian"={"Amplitude"=0.0, "omega(0)"=0.0, "Gamma"=0.0, "phase"=0.0, "Q"=0.0, "Norm  Ampl"=0.0, "z (inf)"=0.0+0.0i, "4corners"={"z (-pi/2)"=0.0+0.0i, "z(inf)"=0.0+0.0i, "z (pi/2)"=0.0+0.0i, "z center"=0.0+0.0i, "z(0)"=0.0+0.0i, "radius"=0.0}}, "timestamp(min)"=1014.5666666701436, "timestamp"=timestamp(3493788695 s since 1904-01-01), "Magn Field(T)"=0.0}, {"temperature"=69.531, "lorentzian"={"Amplitude"=0.0, "omega(0)"=0.0, "Gamma"=0.0, "phase"=0.0, "Q"=0.0, "Norm  Ampl"=0.0, "z (inf)"=0.0+0.0i, "4corners"={"z (-pi/2)"=0.0+0.0i, "z(inf)"=0.0+0.0i, "z (pi/2)"=0.0+0.0i, "z center"=0.0+0.0i, "z(0)"=0.0+0.0i, "radius"=0.0}}, "timestamp(min)"=1015.8833333328366, "timestamp"=timestamp(3493788774 s since 1904-01-01), "Magn Field(T)"=0.0}, {"temperature"=69.468, "lorentzian"={"Amplitude"=0.0, "omega(0)"=0.0, "Gamma"=0.0, "phase"=0.0, "Q"=0.0, "Norm  Ampl"=0.0, "z (inf)"=0.0+0.0i, "4corners"={"z (-pi/2)"=0.0+0.0i, "z(inf)"=0.0+0.0i, "z (pi/2)"=0.0+0.0i, "z center"=0.0+0.0i, "z(0)"=0.0+0.0i, "radius"=0.0}}, "timestamp(min)"=1017.2166666686535, "timestamp"=timestamp(3493788854 s since 1904-01-01), "Magn Field(T)"=0.0}, {"temperature"=69.402, "lorentzian"={"Amplitude"=0.0, "omega(0)"=0.0, "Gamma"=0.0, "phase"=0.0, "Q"=0.0, "Norm  Ampl"=0.0, "z (inf)"=0.0+0.0i, "4corners"={"z (-pi/2)"=0.0+0.0i, "z(inf)"=0.0+0.0i, "z (pi/2)"=0.0+0.0i, "z center"=0.0+0.0i, "z(0)"=0.0+0.0i, "radius"=0.0}}, "timestamp(min)"=1018.5333333313465, "timestamp"=timestamp(3493788933 s since 1904-01-01), "Magn Field(T)"=0.0}, {"temperature"=69.343, "lorentzian"={"Amplitude"=0.0, "omega(0)"=0.0, "Gamma"=0.0, "phase"=0.0, "Q"=0.0, "Norm  Ampl"=0.0, "z (inf)"=0.0+0.0i, "4corners"={"z (-pi/2)"=0.0+0.0i, "z(inf)"=0.0+0.0i, "z (pi/2)"=0.0+0.0i, "z center"=0.0+0.0i, "z(0)"=0.0+0.0i, "radius"=0.0}}, "timestamp(min)"=1019.8666666671634, "timestamp"=timestamp(3493789013 s since 1904-01-01), "Magn Field(T)"=0.0}, {"temperature"=69.279, "lorentzian"={"Amplitude"=0.0, "omega(0)"=0.0, "Gamma"=0.0, "phase"=0.0, "Q"=0.0, "Norm  Ampl"=0.0, "z (inf)"=0.0+0.0i, "4corners"={"z (-pi/2)"=0.0+0.0i, "z(inf)"=0.0+0.0i, "z (pi/2)"=0.0+0.0i, "z center"=0.0+0.0i, "z(0)"=0.0+0.0i, "radius"=0.0}}, "timestamp(min)"=1021.183333337307, "timestamp"=timestamp(3493789092 s since 1904-01-01), "Magn Field(T)"=0.0}, {"temperature"=69.219, "lorentzian"={"Amplitude"=0.0, "omega(0)"=0.0, "Gamma"=0.0, "phase"=0.0, "Q"=0.0, "Norm  Ampl"=0.0, "z (inf)"=0.0+0.0i, "4corners"={"z (-pi/2)"=0.0+0.0i, "z(inf)"=0.0+0.0i, "z (pi/2)"=0.0+0.0i, "z center"=0.0+0.0i, "z(0)"=0.0+0.0i, "radius"=0.0}}, "timestamp(min)"=1022.5, "timestamp"=timestamp(3493789171 s since 1904-01-01), "Magn Field(T)"=0.0}, {"temperature"=69.155, "lorentzian"={"Amplitude"=0.0, "omega(0)"=0.0, "Gamma"=0.0, "phase"=0.0, "Q"=0.0, "Norm  Ampl"=0.0, "z (inf)"=0.0+0.0i, "4corners"={"z (-pi/2)"=0.0+0.0i, "z(inf)"=0.0+0.0i, "z (pi/2)"=0.0+0.0i, "z center"=0.0+0.0i, "z(0)"=0.0+0.0i, "radius"=0.0}}, "timestamp(min)"=1023.8333333358169, "timestamp"=timestamp(3493789251 s since 1904-01-01), "Magn Field(T)"=0.0}, {"temperature"=69.092, "lorentzian"={"Amplitude"=0.0, "omega(0)"=0.0, "Gamma"=0.0, "phase"=0.0, "Q"=0.0, "Norm  Ampl"=0.0, "z (inf)"=0.0+0.0i, "4corners"={"z (-pi/2)"=0.0+0.0i, "z(inf)"=0.0+0.0i, "z (pi/2)"=0.0+0.0i, "z center"=0.0+0.0i, "z(0)"=0.0+0.0i, "radius"=0.0}}, "timestamp(min)"=1025.1499999985099, "timestamp"=timestamp(3493789330 s since 1904-01-01), "Magn Field(T)"=0.0}, {"temperature"=69.033, "lorentzian"={"Amplitude"=0.0, "omega(0)"=0.0, "Gamma"=0.0, "phase"=0.0, "Q"=0.0, "Norm  Ampl"=0.0, "z (inf)"=0.0+0.0i, "4corners"={"z (-pi/2)"=0.0+0.0i, "z(inf)"=0.0+0.0i, "z (pi/2)"=0.0+0.0i, "z center"=0.0+0.0i, "z(0)"=0.0+0.0i, "radius"=0.0}}, "timestamp(min)"=1026.4833333343267, "timestamp"=timestamp(3493789410 s since 1904-01-01), "Magn Field(T)"=0.0}, {"temperature"=68.969, "lorentzian"={"Amplitude"=0.0, "omega(0)"=0.0, "Gamma"=0.0, "phase"=0.0, "Q"=0.0, "Norm  Ampl"=0.0, "z (inf)"=0.0+0.0i, "4corners"={"z (-pi/2)"=0.0+0.0i, "z(inf)"=0.0+0.0i, "z (pi/2)"=0.0+0.0i, "z center"=0.0+0.0i, "z(0)"=0.0+0.0i, "radius"=0.0}}, "timestamp(min)"=1027.8000000044703, "timestamp"=timestamp(3493789489 s since 1904-01-01), "Magn Field(T)"=0.0}, {"temperature"=68.909, "lorentzian"={"Amplitude"=0.0, "omega(0)"=0.0, "Gamma"=0.0, "phase"=0.0, "Q"=0.0, "Norm  Ampl"=0.0, "z (inf)"=0.0+0.0i, "4corners"={"z (-pi/2)"=0.0+0.0i, "z(inf)"=0.0+0.0i, "z (pi/2)"=0.0+0.0i, "z center"=0.0+0.0i, "z(0)"=0.0+0.0i, "radius"=0.0}}, "timestamp(min)"=1029.1166666671634, "timestamp"=timestamp(3493789568 s since 1904-01-01), "Magn Field(T)"=0.0}, {"temperature"=68.845, "lorentzian"={"Amplitude"=0.0, "omega(0)"=0.0, "Gamma"=0.0, "phase"=0.0, "Q"=0.0, "Norm  Ampl"=0.0, "z (inf)"=0.0+0.0i, "4corners"={"z (-pi/2)"=0.0+0.0i, "z(inf)"=0.0+0.0i, "z (pi/2)"=0.0+0.0i, "z center"=0.0+0.0i, "z(0)"=0.0+0.0i, "radius"=0.0}}, "timestamp(min)"=1030.4500000029802, "timestamp"=timestamp(3493789648 s since 1904-01-01), "Magn Field(T)"=0.0}, {"temperature"=68.784, "lorentzian"={"Amplitude"=0.0, "omega(0)"=0.0, "Gamma"=0.0, "phase"=0.0, "Q"=0.0, "Norm  Ampl"=0.0, "z (inf)"=0.0+0.0i, "4corners"={"z (-pi/2)"=0.0+0.0i, "z(inf)"=0.0+0.0i, "z (pi/2)"=0.0+0.0i, "z center"=0.0+0.0i, "z(0)"=0.0+0.0i, "radius"=0.0}}, "timestamp(min)"=1031.7666666656733, "timestamp"=timestamp(3493789727 s since 1904-01-01), "Magn Field(T)"=0.0}, {"temperature"=68.723, "lorentzian"={"Amplitude"=0.0, "omega(0)"=0.0, "Gamma"=0.0, "phase"=0.0, "Q"=0.0, "Norm  Ampl"=0.0, "z (inf)"=0.0+0.0i, "4corners"={"z (-pi/2)"=0.0+0.0i, "z(inf)"=0.0+0.0i, "z (pi/2)"=0.0+0.0i, "z center"=0.0+0.0i, "z(0)"=0.0+0.0i, "radius"=0.0}}, "timestamp(min)"=1033.0833333358169, "timestamp"=timestamp(3493789806 s since 1904-01-01), "Magn Field(T)"=0.0}, {"temperature"=68.661, "lorentzian"={"Amplitude"=0.0, "omega(0)"=0.0, "Gamma"=0.0, "phase"=0.0, "Q"=0.0, "Norm  Ampl"=0.0, "z (inf)"=0.0+0.0i, "4corners"={"z (-pi/2)"=0.0+0.0i, "z(inf)"=0.0+0.0i, "z (pi/2)"=0.0+0.0i, "z center"=0.0+0.0i, "z(0)"=0.0+0.0i, "radius"=0.0}}, "timestamp(min)"=1034.4166666641831, "timestamp"=timestamp(3493789886 s since 1904-01-01), "Magn Field(T)"=0.0}, {"temperature"=68.599, "lorentzian"={"Amplitude"=0.0, 
